vi "fix class control labels.vi"(8 "error in":errorcluster, 10 "class to load":path, 11 "Application in":refnum<vi>) -> (0 "error out":errorcluster)   [LabVIEW 2013, in "NISE Tools Scripting.lvlib"]
uses:
  NISE Tools Scripting.lvlib
  <vilib>/Utility/traverseref.llb/TRef TravTarget.ctl
  <vilib>/Utility/traverseref.llb/VI Scripting - Traverse.lvlib
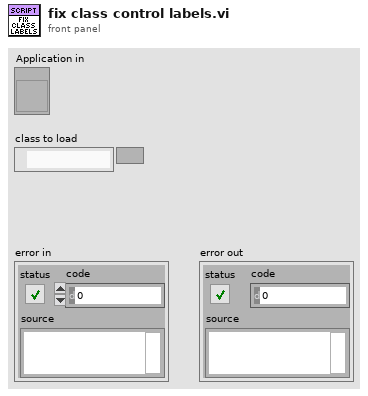
[diagram p1: front panel]
types:
  T1 = typedef "TRef TravTarget.ctl" = enum16{"FP", "BD", "Other"}
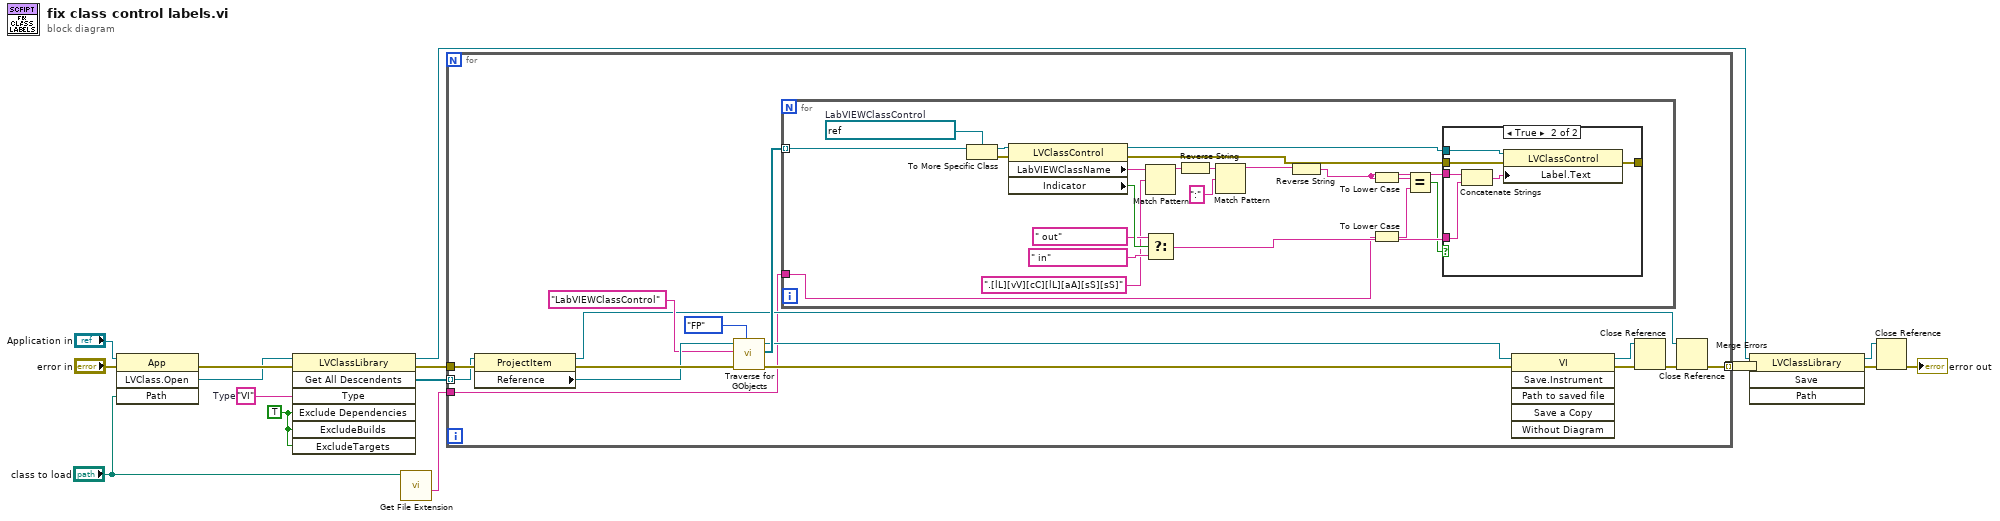
[diagram p0: block diagram]
diagram:
  w12 = TRUE
  w11 = "VI"  # Type
  n1 = invoke class="App" method="LVClass.Open"(reference="Application in", error in="error in", "Path"="class to load") -> (error out=w13:errorcluster, "LVClass.Open"=w10:refnum<vi>)  [unwired: 1 in, 2 out]
  n2 = invoke class="LVClassLibrary" method="Get All Descendents"(reference=w10, error in=w13, "Type"=w11, "Exclude Dependencies"=w12, "ExcludeBuilds"=w12, "ExcludeTargets"=w12) -> (reference out=w8:refnum<vi>, error out=w15:errorcluster, "All Descendents"=w14:refnum<vi>[])  [unwired: 1 in, 4 out]
  n3 = call <vilib>:"Get File Extension.vi"("file"="class to load") -> ("filename without extension"=w2:string)  [unwired: 7 in, 3 out]
  n4 = for {
    tunnel: w14 -> [w30] mode=indexing
    tunnel: w2 -> [w17]
    tunnel: w15 -> [w31]
    tunnel: [w22] -> w16 mode=indexing
    n5 = property class="ProjectItem"(reference=w30, error in=w31) -> (reference out=w21:refnum<vi>, error out=w29:errorcluster, "Reference"=w28:refnum<vi>)
    n6 = call <vilib>:"Traverse for GObjects.vi"("Traverse Target"=TRef_TravTarget."FP", "error in (no error)"=w29, "Class Name"="LabVIEWClassControl", "VI Refnum"=w28) -> ("error out"=w18:errorcluster, "References"=w25:refnum<vi>[], "dup VI Refnum"=w24:refnum<vi>)  [unwired: 4 in, 1 out]
    n7 = for {
      tunnel: w25 -> [w51] mode=indexing
      tunnel: w17 -> [w40]
      w49 = refnum<vi> refnum  # LabVIEWClassControl
      n8 = To More Specific Class(target class=w49, reference=w51) -> (specific class reference=w50:refnum<vi>, error out=w52:errorcluster)  [unwired: 1 in]
      n9 = property class="LVClassControl"(reference=w50, error in=w52) -> (reference out=w48:refnum<vi>, error out=w47:errorcluster, "LabVIEWClassName"=w42:string, "Indicator"=w46:bool)
      n10 = Match Pattern(string=w42, regular expression=".[lL][vV][cC][lL][aA][sS][sS]") -> (before substring=w35:string)  [unwired: 1 in, 3 out]
      n11 = Select(t=" out", s=w46, f=" in") -> (s? t:f=w43:string)
      n12 = Reverse String(1:w35) -> (0:w34:string)
      n13 = Match Pattern(string=w34, regular expression=":") -> (before substring=w33:string)  [unwired: 1 in, 3 out]
      n14 = Reverse String(1:w33) -> (0:w32:string)
      n15 = To Lower Case(string=w32) -> (all lower case string=w38:string)
      n16 = To Lower Case(string=w40) -> (all lower case string=w39:string)
      n17 = Equal?(x=w38, y=w39) -> (x = y?=w37:bool)
      n18 = case shown="True" w37 {
        tunnel: w48 -> [_ w59]
        tunnel: w47 -> [w53 w58]
        tunnel: w43 -> [_ w56]
        tunnel: [w53 w55] -> _
        tunnel: w32 -> [_ w54]
        frame False {
        }
        frame True {
          n19 = Concatenate Strings(w54, w56) -> (w57:string)
          n20 = property class="LVClassControl"(reference=w59, error in=w58, "Label.Text"=w57) -> (error out=w55:errorcluster)  [unwired: 1 out]
        }
      }
    }
    n21 = invoke class="VI" method="Save.Instrument"(reference=w24, error in=w18) -> (reference out=w19:refnum<vi>, error out=w20:errorcluster)  [unwired: 4 in, 4 out]
    n22 = Close Reference(reference=w19, error in (no error)=w20) -> (error out=w23:errorcluster)
    n23 = Close Reference(reference=w21, error in (no error)=w23) -> (error out=w22:errorcluster)
  }
  n24 = Merge Errors(w16) -> (w1:errorcluster)
  n25 = invoke class="LVClassLibrary" method="Save"(reference=w8, error in=w1) -> (reference out=w7:refnum<vi>, error out=w9:errorcluster)  [unwired: 2 in, 2 out]
  n26 = Close Reference(reference=w7, error in (no error)=w9) -> (error out=→"error out":errorcluster)
